vi "Write Laser Controller.vi"(8 "error in (no error)":errorcluster, 10 "Laser Controller.lvclass":refnum<class "Laser Controller.lvclass">, 11 "Laser View in":refnum<class "Laser View.lvclass">) -> (0 "error out":errorcluster, 3 "Laser View out":refnum<class "Laser View.lvclass">)   [LabVIEW 2022 SP3]
uses:
  Laser View.lvclass
  Laser Controller/Laser Controller.lvclass
  Laser View.lvclass/Laser View.ctl
  C:/XY Stage/iView/base view/base view.lvclass
  C:/XY Stage/iView/iView/iView.lvclass
  C:/XY Stage/Laser/Laser View/Laser View.lvclass
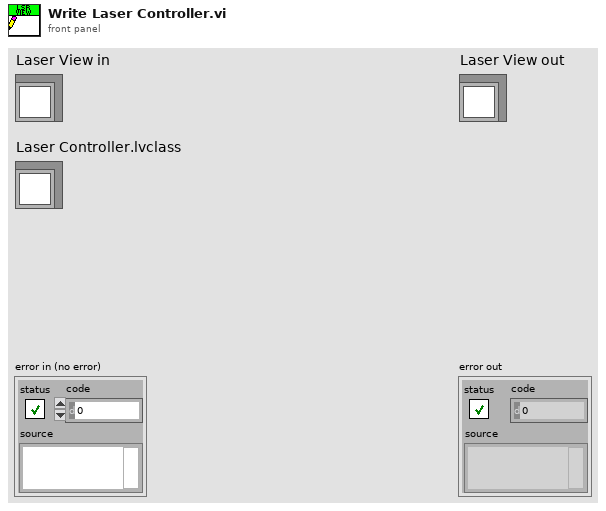
[diagram p1: front panel]
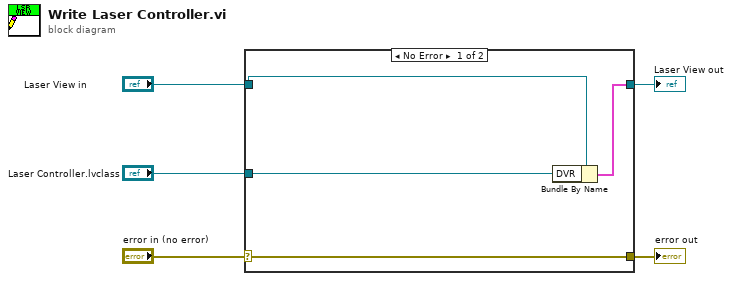
[diagram p0: block diagram]
diagram:
  n1 = case shown="No Error" "error in (no error)" {
    selector: "error in (no error)" -> [w9 w10]
    tunnel: [w9 w10] -> w4
    tunnel: [w7 w11] -> w2
    tunnel: "Laser View in" -> [w8 w11]
    tunnel: "Laser Controller.lvclass" -> [w6 _]
    frame No Error {
      n2 = Bundle By Name(cluster=w8, "DVR"=w6) -> (w7:cluster{})
    }
    frame Error {
    }
  }
  "error out" <- w4
  "Laser View out" <- w2
